vi "Set Max. Speed.vi"(8 "error in (no error)":errorcluster, 10 "XYZ Position Input":T1={"Speed"=0, "Z Limit (um+/-)"=0.0, "Axes"="Z", "XYZ Coordinates"={"X"=0.0, "Y"=0.0, "Z"=0.0}} {"XYZ Coordinates"."Z" format="Z= %#_g"; "XYZ Coordinates"."Y" format="Y= %#_g"; "XYZ Coordinates"."X" format="X= %#_g"; "Z Limit (um+/-)" format="Z Limit = %.0f"; "Speed" format="Speed= %.0f"}, 11 "Scientifica XYZ Gen1 in":refnum<class "Scientifica XYZ Gen1.lvclass">) -> (0 "error out":errorcluster, 2 "read string":string, 3 "Scientifica XYZ Gen1 out":refnum<class "Scientifica XYZ Gen1.lvclass">)   [LabVIEW 2020, in "TranslationStageClassStructure.lvlib" / "Scientifica XYZ Gen1.lvclass"]
uses:
  Scientifica XYZ Gen1.lvclass
  XYZ Stage Control/typedefs/XYZ_position_input.ctl
  XYZ Stage Control/typedefs/XYZ axes.ctl
  Typedefs/XYZ_coordinates.ctl
  Scientifica XYZ Gen1.lvclass/Scientifica XYZ Gen1.ctl
  Serial Comms/Serial Comms/Serial Comms.lvclass
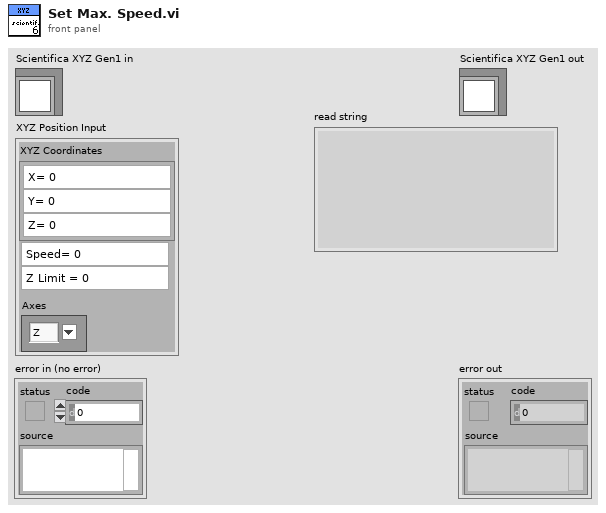
[diagram p1: front panel]
types:
  T1 = typedef "XYZ_position_input.ctl" = cluster{"Speed":i32, "Z Limit (um+/-)":sgl, "Axes":T2, "XYZ Coordinates":T3}
  T2 = typedef "XYZ axes.ctl" = string
  T3 = typedef "XYZ_coordinates.ctl" = cluster{"X":sgl, "Y":sgl, "Z":sgl}
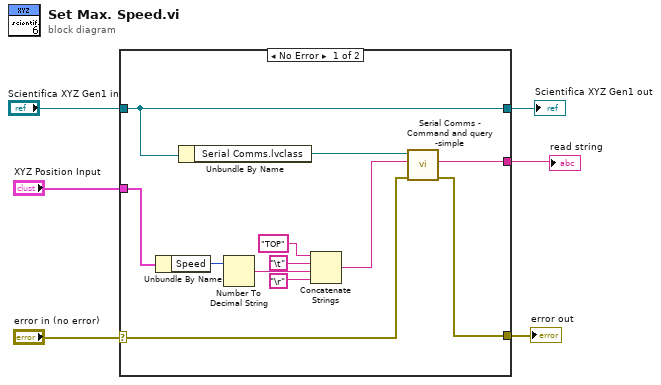
[diagram p0: block diagram]
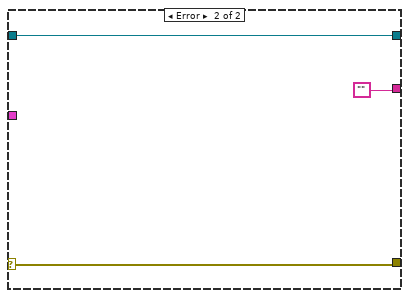
[diagram p2: hidden frame]
diagram:
  n1 = case shown="No Error" "error in (no error)" {
    selector: "error in (no error)" -> [w16 w20]
    tunnel: "Scientifica XYZ Gen1 in" -> [w17 w21]
    tunnel: [w17 w21] -> w4
    tunnel: [w15 w20] -> w3
    tunnel: "XYZ Position Input" -> [w8 _]
    tunnel: [w7 ""] -> w1
    frame No Error {
      n2 = Unbundle By Name(w8) -> ("Speed"=w10:i32)
      n3 = Unbundle By Name(w17) -> ("Serial Comms.lvclass"=w18:refnum<class "Serial Comms.lvclass">)
      n4 = Number To Decimal String(number=w10) -> (decimal integer string=w14:string)  [unwired: 1 in]
      n5 = Concatenate Strings("TOP" ("decimal integer string"), "\t" ("Tab Constant"), w14, "\r" ("Carriage Return Constant")) -> (w9:string)
      n6 = call "Serial Comms - Command and query -simple.vi"("error in (no error)"=w16, "string to write"=w9, "Serial Comms in"=w18) -> ("error out"=w15:errorcluster, "read string"=w7:string)  [unwired: 4 in, 3 out]
    }
    frame Error {
    }
  }
  "error out" <- w3
  "Scientifica XYZ Gen1 out" <- w4
  "read string" <- w1
